vi "XIPIN_AXI4-Stream_to_Video_Out_2_01_a.vi"   [LabVIEW 2017]
doc: "Bridge from AXI4-Stream slave bus to video output with syncs.\n------------------------------------\n<b>Need License</b> : No\n<b>Interface</b> : AXI4-Stream"
uses:
  <vilib>/rvi/XilinxIP/XIPIN_XNode/niFpgaXIPIN.xnode
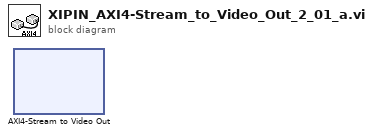
[diagram p0: block diagram]
diagram:
  n1 = xnode ("AXI4-Stream to Video Out")() -> ()
